vi "Do.vi"(8 "error in (no error)":errorcluster, 10 "Actor in":refnum<class "Actor.lvclass">, 11 "TCP-SV Message Interpreter Msg":refnum<class "TCP-SV Message Interpreter Msg.lvclass">) -> (0 "error out":errorcluster, 2 "Actor out":refnum<class "Actor.lvclass">)   [LabVIEW 2026, in "TALOS.lvlib" / "Guardian.lvlib" / "TCP-SV Message Interpreter Msg.lvclass"]
doc: "This VI delivers the message to the actor by calling the appropriate method(s) on the actor."
uses:
  TCP-SV Message Interpreter Msg.lvclass
  builds/Actor Framework PPL/Actor Framework.lvlibp/1abvi3w/vi.lib/ActorFramework/Actor/Actor.lvclass
  TCP-SV Message Interpreter Msg.lvclass/TCP-SV Message Interpreter Msg.ctl
  Guardian/Guardian.lvclass
  C:/LabVIEW Code/TALOS/builds/Actor Framework PPL/Actor Framework.lvlibp/1abvi3w/vi.lib/ActorFramework/Actor/Actor.lvclass
  7835297c-3f2a-42c5-bff3-3fa71d0bcaf8.vi
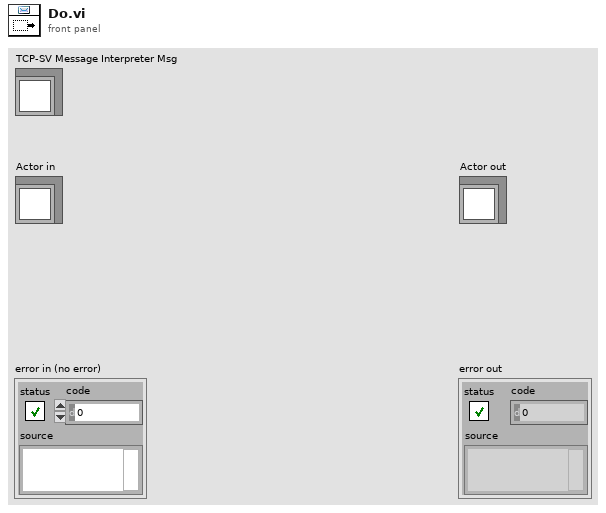
[diagram p1: front panel]
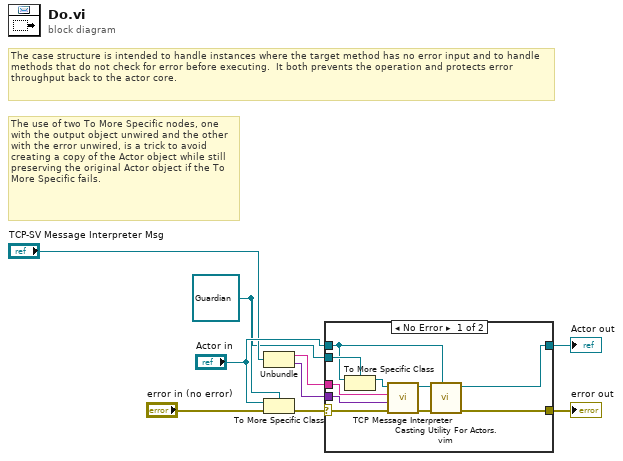
[diagram p0: block diagram]
diagram:
  w4 = refnum<class "Guardian.lvclass"> refnum ("Actor in")
  # "The use of two To More Specific nodes, one with the output object unwired and the other with the error unwired, is a trick to avoid creating a copy of the Actor object while still preserving the original Actor object if the To More Specific fails."
  # "The case structure is intended to handle instances where the target method has no error input and to handle methods that do not check for error before executing.  It both prevents the operation and protects error throughput back to the actor core."
  n1 = Unbundle("TCP-SV Message Interpreter Msg") -> (w2:string, w1:variant)
  n2 = To More Specific Class(target class=w4, reference="Actor in", error in="error in (no error)") -> (error out=w3:errorcluster)  [unwired: 1 out]
  n3 = case shown="No Error" w3 {
    selector: w3 -> [w19 w21]
    tunnel: [w13 w21] -> w9
    tunnel: [w14 w20] -> w8
    tunnel: "Actor in" -> [w16 w20]
    tunnel: w4 -> [w17 _]
    tunnel: w2 -> [w11 _]
    tunnel: w1 -> [w10 _]
    frame No Error {
      n4 = To More Specific Class(target class=w17, reference=w16) -> (specific class reference=w18:refnum<class "Guardian.lvclass">)  [unwired: 1 in, 1 out]
      n5 = call "TCP Message Interpreter.vi"("error in (no error)"=w19, "Data"=w10, "Message"=w11, "Guardian in"=w18) -> ("error out"=w12:errorcluster, "Guardian out"=w15:refnum<class "Guardian.lvclass">)  [unwired: 6 in]
      n6 = call "Casting Utility For Actors.vim"("type"=w16, "error in (no error)"=w12, "Actor in"=w15) -> ("error out"=w13:errorcluster, "Actor out"=w14:refnum<class "Actor.lvclass">)  [unwired: 7 in]
    }
    frame Error {
      # "If type check fails, pass the original object out again."
    }
  }
  "error out" <- w9
  "Actor out" <- w8
